vi "file matching.vi"() -> ()   [LabVIEW 2014]
uses:
  <vilib>/regexp/Match Regular Expression.xnode
panel:
  out "the field of interest":string[][](array[string])
  out "target port":string[](array[string])
  out "source port":string[](array[string])
  out "target ip":string[](array[string])
  out "source ip":string[](array[string])
  out "length":string[](array[string])
  out "Protocol":string[](array[string])
  out "block / pass":string[](array[string])
  out "Interface name":string[](array[string])
  out "Date time":string[](array[string])
  in  "String":string
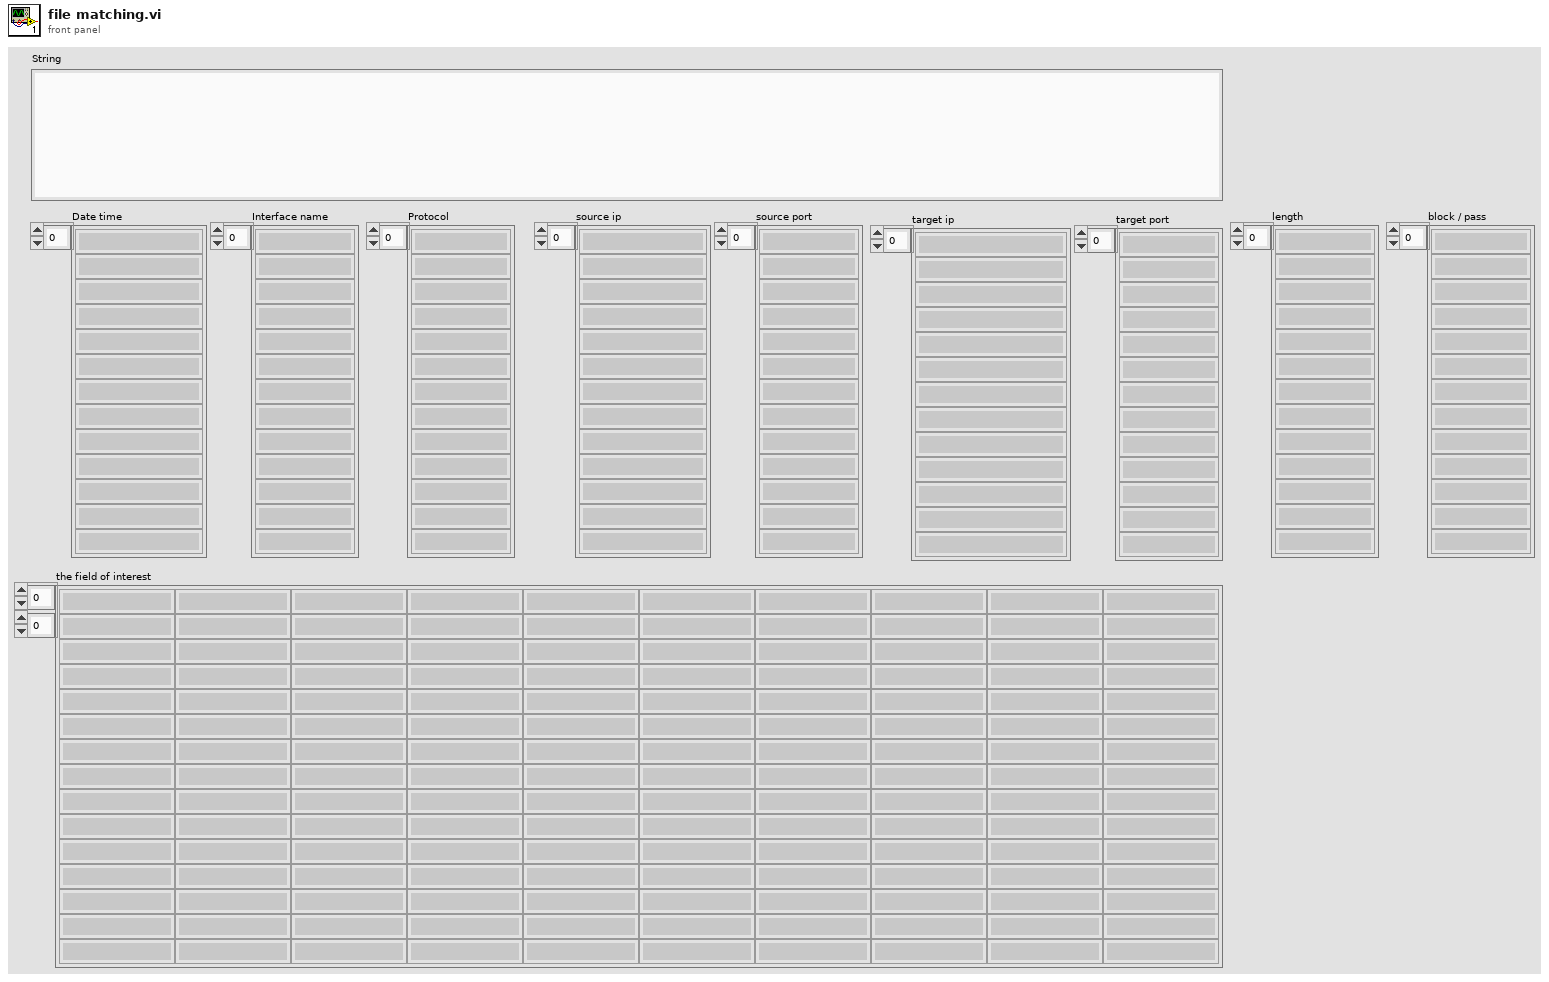
[diagram p1: front panel]
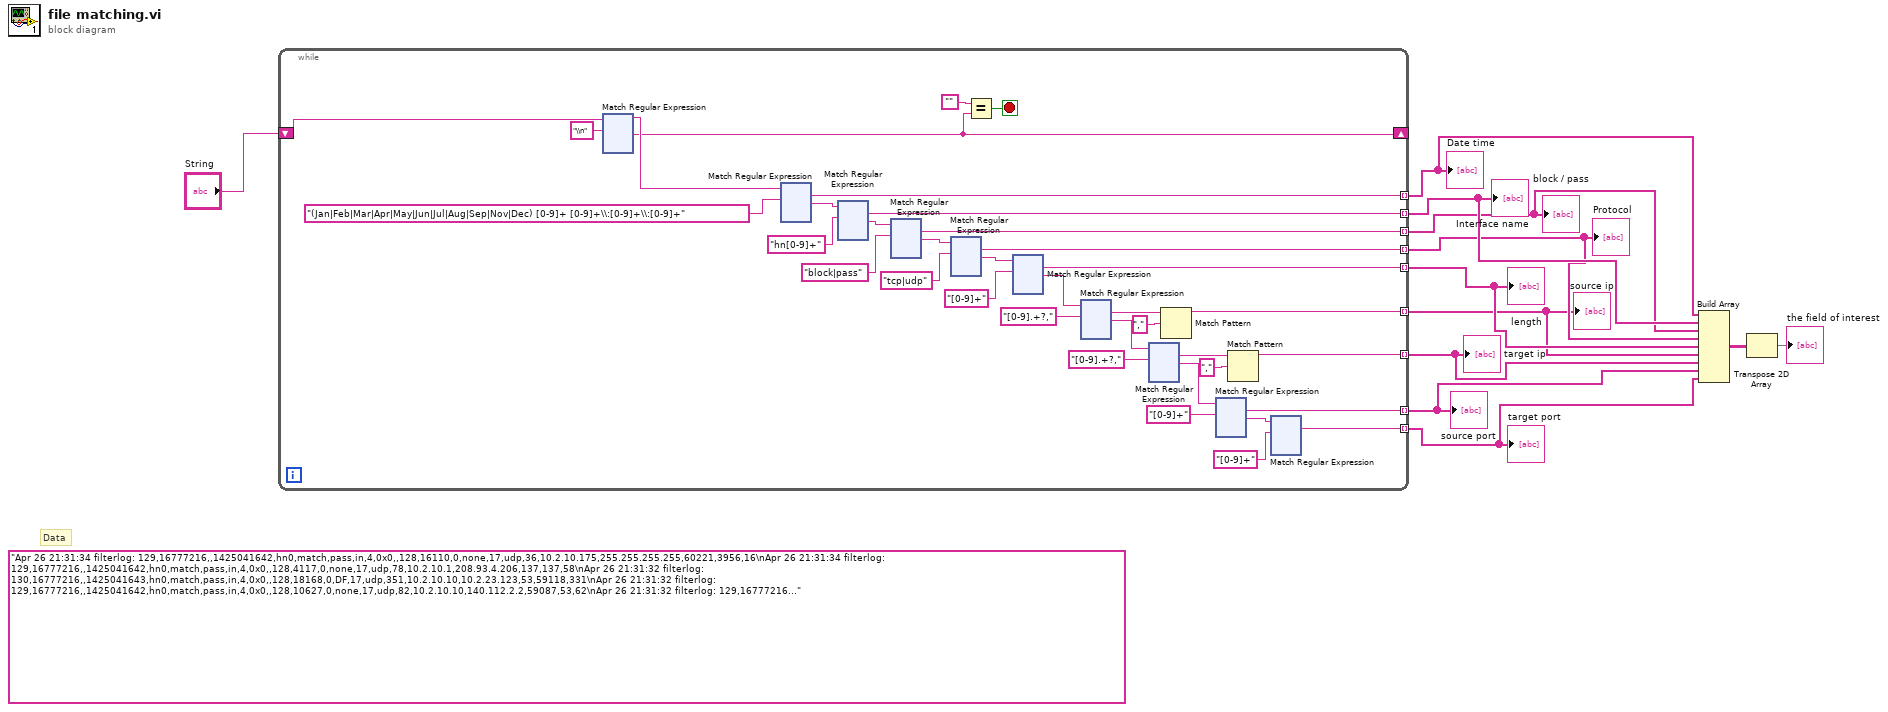
[diagram p0: block diagram]
diagram:
  (unwired) "Apr 26 21:31:34 filterlog: 129,16777216,,1425041642,hn0,match,pass,in,4,0x0,,128,16110,0,none,17,udp,36,10.2.10.175,255.255.255.255,60221,3956,16\nApr 26 21:31:34 filterlog: 129,16777216,,1425041642,hn0,match,pass,in,4,0x0,,128,4117,0,none,17,udp,78,10.2.10.1,208.93.4.206,137,137,58\nApr 26 21:31:32 filterlog: 130,16777216,,1425041643,hn0,match,pass,in,4,0x0,,128,18168,0,DF,17,udp,351,10.2.10.10,10.2.23.123,53,59118,331\nApr 26 21:31:32 filterlog: 129,16777216,,1425041642,hn0,match,pass,in,4,0x0,,128,10627,0,none,17,udp,82,10.2.10.10,140.112.2.2,59087,53,62\nApr 26 21:31:32 filterlog: 129,16777216,,1425041642,hn0,match,pass,in,4,0x0,,128,10626,0,none,17,udp,98,10.2.10.10,140.112.2.2,60847,53,78\nApr 26 21:38:10 filterlog: 105,16777216,,1425041627,hn1,match,block,in,4,0x2,0,109,9812,0,DF,6,tcp,48,207.46.13.171,10.2.10.15,25309,80,0,SEC,27892632,,8192,,mss;nop;nop;sackOK\nApr 26 21:38:08 filterlog: 129,16777216,,1425041642,hn0,match,pass,in,4,0x0,,128,23124,0,DF,6,tcp,52,10.2.10.172,207.46.153.155,60590,443,0,S,2141064781,,8192,,mss;nop;wscale;nop;nop;sackOK\nApr 26 21:38:08 filterlog: 130,16777216,,1425041643,hn0,match,block,in,4,0x2,0,128,8596,0,DF,6,tcp,48,10.2.10.2,10.2.102.10,41875,88,0,SEC,3256166066,,8192,,mss;nop;nop;sackOK\nApr 26 21:38:07 filterlog: 130,16777216,,1425041643,hn0,match,pass,in,4,0x2,0,128,8592,0,DF,6,tcp,48,10.2.10.2,10.2.102.10,41874,88,0,SEC,2184502132,,8192,,mss;nop;nop;sackOK\n"
  # "Data"
  n1 = while {
    tunnel: [w27] -> w11 mode=indexing
    tunnel: [w26] -> w10 mode=indexing
    tunnel: [w25] -> w9 mode=indexing
    tunnel: [w24] -> w8 mode=indexing
    tunnel: [w23] -> w7 mode=indexing
    tunnel: [w22] -> w6 mode=indexing
    tunnel: [w21] -> w5 mode=indexing
    tunnel: [w20] -> w4 mode=indexing
    tunnel: [w19] -> w3 mode=indexing
    shift-right: [w13] -> _
    shift-left: "String" -> [w15]
    stop <- w18 stop-if-true
    n2 = xnode "Match Regular Expression"("input string"=w15, "regular expression"="\\n") -> ("before match"=w14:string, "after match"=w13:string)  [unwired: 4 in, 3 out]
    n3 = xnode "Match Regular Expression"("input string"=w14, "regular expression"="(Jan|Feb|Mar|Apr|May|Jun|Jul|Aug|Sep|Nov|Dec) [0-9]+ [0-9]+\\:[0-9]+\\:[0-9]+") -> ("whole match"=w27:string, "after match"=w47:string)  [unwired: 4 in, 3 out]
    n4 = xnode "Match Regular Expression"("input string"=w47, "regular expression"="hn[0-9]+") -> ("whole match"=w26:string, "after match"=w45:string)  [unwired: 4 in, 3 out]
    n5 = xnode "Match Regular Expression"("input string"=w45, "regular expression"="block|pass") -> ("whole match"=w25:string, "after match"=w43:string)  [unwired: 4 in, 3 out]
    n6 = xnode "Match Regular Expression"("input string"=w43, "regular expression"="tcp|udp") -> ("whole match"=w24:string, "after match"=w41:string)  [unwired: 4 in, 3 out]
    n7 = Equal?(x="", y=w13) -> (x = y?=w18:bool)
    n8 = xnode "Match Regular Expression"("input string"=w41, "regular expression"="[0-9]+") -> ("whole match"=w23:string, "after match"=w39:string)  [unwired: 4 in, 3 out]
    n9 = xnode "Match Regular Expression"("input string"=w39, "regular expression"="[0-9].+?,") -> ("whole match"=w31:string, "after match"=w37:string)  [unwired: 4 in, 3 out]
    n10 = xnode "Match Regular Expression"("input string"=w37, "regular expression"="[0-9].+?,") -> ("whole match"=w28:string, "after match"=w35:string)  [unwired: 4 in, 3 out]
    n11 = Match Pattern(string=w31, regular expression=",") -> (before substring=w22:string)  [unwired: 1 in, 3 out]
    n12 = xnode "Match Regular Expression"("input string"=w35, "regular expression"="[0-9]+") -> ("whole match"=w20:string, "after match"=w33:string)  [unwired: 4 in, 3 out]
    n13 = Match Pattern(string=w28, regular expression=",") -> (before substring=w21:string)  [unwired: 1 in, 3 out]
    n14 = xnode "Match Regular Expression"("input string"=w33, "regular expression"="[0-9]+") -> ("whole match"=w19:string)  [unwired: 4 in, 4 out]
  }
  "Date time" <- w11
  "Interface name" <- w10
  "block / pass" <- w9
  "Protocol" <- w8
  "length" <- w7
  "source ip" <- w6
  "target ip" <- w5
  "source port" <- w4
  "target port" <- w3
  n15 = Build Array(w11, w10, w9, w8, w7, w6, w5, w4, w3) -> (w2:string[][])
  n16 = Transpose 2D Array(2D array=w2) -> (transposed array=→"the field of interest":string[][])
